vi "Status Channel Summary Query.vi"(0 "VISA resource name":refnum<visa-resource-name>, 7 "Query Reg (F:Summary Enable)":bool, 11 "error in (no error)":errorcluster) -> (4 "VISA resource name out":refnum<visa-resource-name>, 8 "Channel Sum Reg (CH1-8 F:0)":T1, 15 "error out":errorcluster)   [LabVIEW 2015, in "Chroma ATE 6310.lvlib"]
doc: "The VI returns the value of the Channel Summary Enable register or the Channel Summary Event register.\n\nThe Channel Summary Event register indicates all channels on which an enable event has occurred since last time the register was read.Reading this register resets it to zero.\n\nThe Channel Summary Enable register enables channel."
uses:
  <instrlib>/Chroma ATE 6310/Chroma ATE 6310.lvlib
panel:
  # "Event\nSummary Enable"
  # "Channel :       1          2          3          4           5          6          7          8"
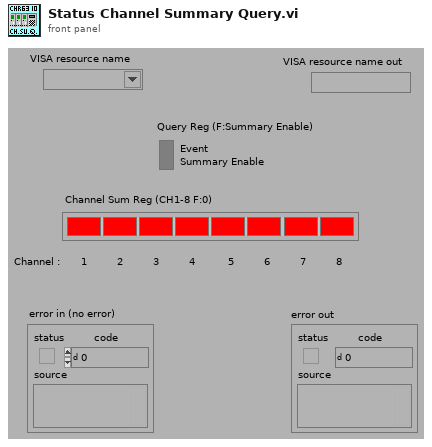
[diagram p1: front panel]
types:
  T1 = cluster{"CH1 (F:0)":bool, "CH2 (F:0)":bool, "CH3 (F:0)":bool, "CH4 (F:0)":bool, "CH5 (F:0)":bool, "CH6 (F:0)":bool, "CH7 (F:0)":bool, "CH8 (F:0)":bool}
  T2 = cluster{"[0]":bool, "[1]":bool, "[2]":bool, "[3]":bool, "[4]":bool, "[5]":bool, "[6]":bool, "[7]":bool}
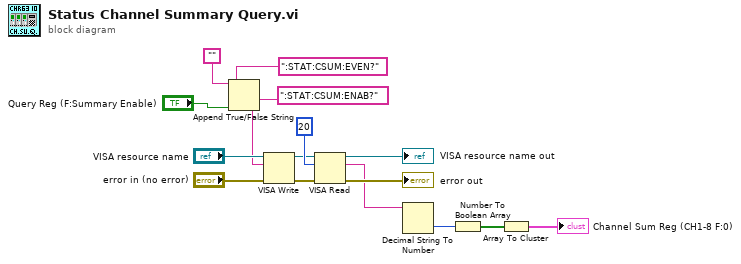
[diagram p0: block diagram]
diagram:
  n1 = Append True/False String(1:"Query Reg (F:Summary Enable)", 2:":STAT:CSUM:ENAB?", 3:":STAT:CSUM:EVEN?", 4:"") -> (0:w8:string)
  n2 = VISA Write(VISA resource name="VISA resource name", write buffer=w8, error in (no error)="error in (no error)") -> (VISA resource name out=w15:refnum<visa-resource-name>, error out=w14:errorcluster)  [unwired: 1 out]
  n3 = VISA Read(VISA resource name=w15, byte count=20, error in (no error)=w14) -> (VISA resource name out=→"VISA resource name out":refnum<visa-resource-name>, read buffer=w4:string, error out=→"error out":errorcluster)  [unwired: 1 out]
  n4 = Decimal String To Number(string=w4) -> (number=w2:i32)  [unwired: 2 in, 1 out]
  n5 = Number To Boolean Array(number=w2) -> (Boolean array=w3:bool[])
  n6 = Array To Cluster(array=w3) -> (cluster=→"Channel Sum Reg (CH1-8 F:0)":T2)
